vi "Timestamp_Conversion.vi"() -> ()   [LabVIEW 2015]
uses:
  <vilib>/Utility/miscctls.llb/LVDateTimeRec.ctl
panel:
  out "Time Stamp UTC":timestamp
  out "Time Stamp Locale":timestamp
  in  "Locale Time Stamp":timestamp=timestamp(3357626462.919444 s since 1904-01-01)
  out "Time Stamp Locale":timestamp
  out "Time Stamp UTC":timestamp
  in  "UTC Time Stamp":timestamp=timestamp(3357626462.919444 s since 1904-01-01)
  out "Locale time zone":string
  out "Difference between UTC and locale":string
  out "UTC Current Time":string
  out "Locale Current Time":string
  # "Use this VI example to understand methods for inter-changing timestamps\nbetween Locale and UTC.\nNote: The Time Stamp format does not contain locale information and\nmust be interpreted as UTC or Locale as appropriate.\nNote: Daylight Savings Time (DST) is automatically considered as a part of the\nLocale settings\nNote: Changes to the Windows Time Zone settings will only be recognised\nby LabVIEW following a restart."
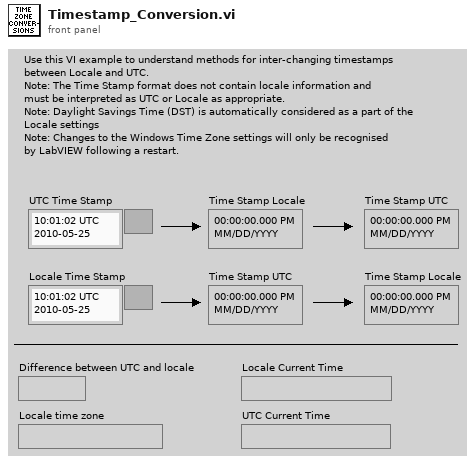
[diagram p1: front panel]
types:
  T1 = typedef "LVDateTimeRec.ctl" = cluster{"fractional second":dbl, "second":i32, "minute":i32, "hour":i32, "day of month":i32, "month":i32, "year":i32, "day of week":i32, "day of year":i32, "DST":i32}
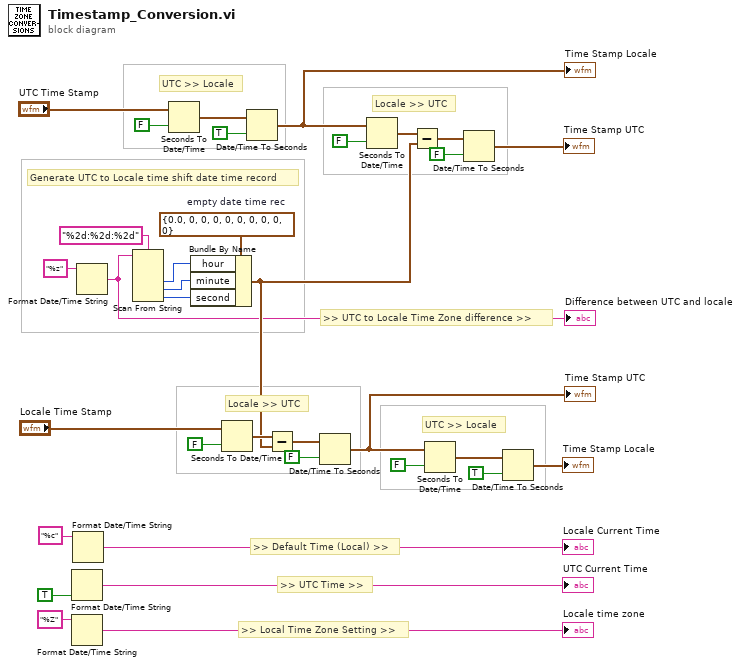
[diagram p0: block diagram]
diagram:
  w19 = T1 {"fractional second"=0.0, "second"=0, "minute"=0, "hour"=0, "day of month"=0, "month"=0, "year"=0, "day of week"=0, "day of year"=0, "DST"=0}  # empty date time rec
  # "Generate UTC to Locale time shift date time record"
  # ">> UTC to Locale Time Zone difference >>"
  # ">> Local Time Zone Setting >>"
  # ">> UTC Time >>"
  # ">> Default Time (Local) >>"
  # "Locale >> UTC"
  # "Locale >> UTC"
  # "UTC >> Locale"
  # "UTC >> Locale"
  n1 = Format Date/Time String(UTC format=TRUE) -> (date/time string=→"UTC Current Time":string)  [unwired: 2 in]
  n2 = Format Date/Time String(time format string (%c)="%Z") -> (date/time string=→"Locale time zone":string)  [unwired: 2 in]
  n3 = Format Date/Time String(time format string (%c)="%c") -> (date/time string=→"Locale Current Time":string)  [unwired: 2 in]
  n4 = Format Date/Time String(time format string (%c)="%z") -> (date/time string=w1:string)  [unwired: 2 in]
  "Difference between UTC and locale" <- w1
  n5 = Scan From String(format string="%2d:%2d:%2d", input string=w1) -> (output 1=w18:i32, output 2=w17:i32, output 3=w16:i32)  [unwired: 5 in, 3 out]
  n6 = Seconds To Date/Time(time stamp (now)="UTC Time Stamp", to UTC (F)=FALSE) -> (date time rec=w15:T1)
  n7 = Bundle By Name(cluster=w19, "hour"=w18, "minute"=w17, "second"=w16) -> (w3:T1)
  n8 = Seconds To Date/Time(time stamp (now)="Locale Time Stamp", to UTC (F)=FALSE) -> (date time rec=w8:T1)
  n9 = Date/Time To Seconds(1:TRUE ("is UTC (F)"), 2:w15) -> (0:w11:timestamp)
  "Time Stamp Locale" <- w11
  n10 = Subtract(x=w8, y=w3) -> (x-y=w6:T1)
  n11 = Date/Time To Seconds(1:FALSE ("is UTC (F)"), 2:w6) -> (0:w2:timestamp)
  "Time Stamp UTC" <- w2
  n12 = Seconds To Date/Time(time stamp (now)=w11, to UTC (F)=FALSE) -> (date time rec=w10:T1)
  n13 = Subtract(x=w10, y=w3) -> (x-y=w13:T1)
  n14 = Seconds To Date/Time(time stamp (now)=w2, to UTC (F)=FALSE) -> (date time rec=w24:T1)
  n15 = Date/Time To Seconds(1:FALSE ("is UTC (F)"), 2:w13) -> (0:→"Time Stamp UTC":timestamp)
  n16 = Date/Time To Seconds(1:TRUE ("is UTC (F)"), 2:w24) -> (0:→"Time Stamp Locale":timestamp)
